vi "Keithley 2002 Multi Read.vi"(0 "GPIB address":string="16", 1 "delay (secs)":dbl min=0.0 max=999999.999 format="%.3f", 2 "source (imm:1)":u16(ring)=1 items=["hold", "immediate", "timer", "manual", "bus", "trigger link", "external"], 3 "timer value (secs)":dbl=0.001 min=0.001 max=999999.999 format="%.3f", 4 "count value":dbl=10.0 min=2.0 max=30092.0 step=1.0, 5 "error in":T2, 7 "delay between\nbus triggers (mS)":dbl=300.0 min=0.0 step=1.0) -> (6 "measurements":T1(array[cluster]) {"measurement" format="%.6e"}, 8 "error out":T2)   [LabVIEW 2020]
doc: "This VI is used to control the Measure Layer (Trigger) settings and then read back the specified number of readings.\n\nThe function of the instrument will not be changed. To take measurements for a new function, you must first configure the instrument with that function's VI.\n\nThe element of the array that stores readings is always 1 number less than the reading number. For example, the array starts at the number 0, while the readings start at 1."
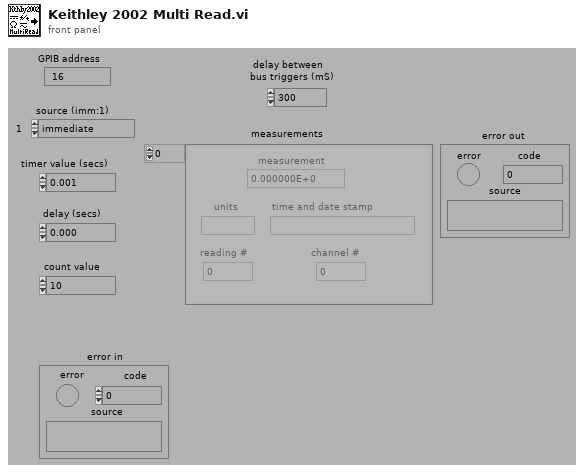
[diagram p1: front panel]
types:
  T1 = cluster{"measurement":dbl, "units":string, "time and date stamp":string, "reading #":dbl, "channel #":dbl}[]
  T2 = cluster{"error":bool, "code":i32, "source":string}
  T3 = cluster{dbl, "read buffer":string, "read buffer":string, dbl, dbl}
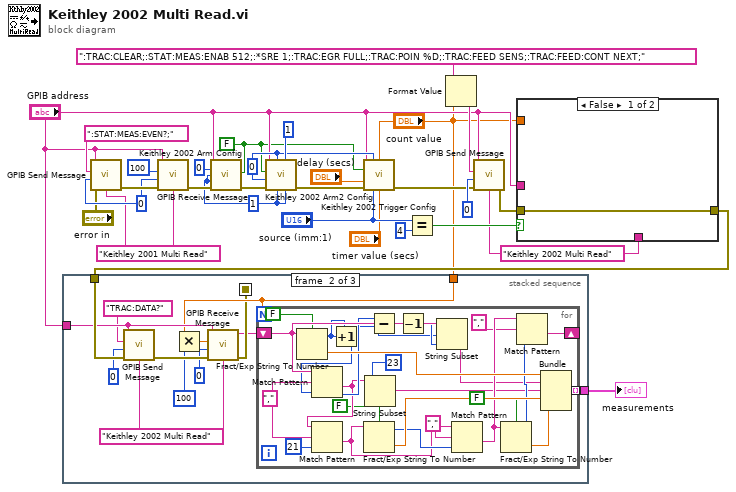
[diagram p0: block diagram]
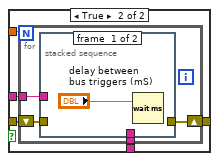
[diagram p2: hidden frame]
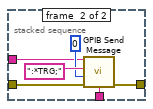
[diagram p3: hidden frame]
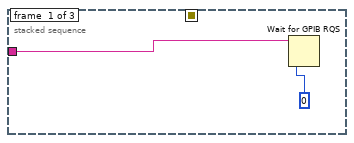
[diagram p4: hidden frame]
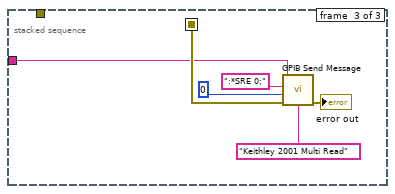
[diagram p5: hidden frame]
diagram:
  w18 = "Keithley 2001 Multi Read"
  w24 = 0
  w7 = 0
  w5 = FALSE
  w3 = 1
  w20 = "Keithley 2002 Multi Read"
  n1 = call "GPIB Send Message.vi"("address string"="GPIB address", "write buffer"=":STAT:MEAS:EVEN?;", "source"=w18, "write mode (set END:0)"=w24, "error in"="error in") -> ("error out"=w27:T2)  [unwired: 2 in, 2 out]
  n2 = call "GPIB Receive Message.vi"("address string"="GPIB address", "byte count"=100, "source"=w18, "read mode"=w24, "error in"=w27) -> ("error out"=w15:T2)  [unwired: 2 in, 2 out]
  n3 = call "Keithley 2002 Arm Config.vi"("GPIB address"="GPIB address", "count (set:0)"=0, "count value"=w3, "direction"=w5, "source (imm:1)"=w3, "error in"=w15) -> ("error out"=w14:T2)  [unwired: 9 in]
  n4 = call "Keithley 2002 Arm2 Config.vi"("timer value (secs)"=w3, "count value"=1, "source (imm:1)"=w3, "count (set:0)"=w7, "error in"=w14, "delay (secs)"=w7, "direction"=w5, "GPIB address"="GPIB address") -> ("error out"=w13:T2)  [unwired: 3 in]
  n5 = call "Keithley 2002 Trigger Config.vi"("GPIB address"="GPIB address", "count (set:0)"=w7, "count value"="count value", "direction"=w5, "delay (secs)"="delay (secs)", "error in"=w13, "source (imm:1)"="source (imm:1)", "timer value (secs)"="timer value (secs)") -> ("error out"=w12:T2)  [unwired: 7 in]
  n6 = Equal?(x="source (imm:1)", y=4) -> (x = y?=w21:bool)
  n7 = Format Value(format string=":TRAC:CLEAR;:STAT:MEAS:ENAB 512;:*SRE 1;:TRAC:EGR FULL;:TRAC:POIN %D;:TRAC:FEED SENS;:TRAC:FEED:CONT NEXT;", value (0)="count value") -> (output string=w16:string)  [unwired: 1 in]
  n8 = call "GPIB Send Message.vi"("address string"="GPIB address", "write buffer"=w16, "source"=w20, "write mode (set END:0)"=0, "error in"=w12) -> ("error out"=w22:T2)  [unwired: 2 in, 2 out]
  n9 = case shown="False" w21 {
    tunnel: [w30 w35] -> w19
    tunnel: w20 -> [_ w34]
    tunnel: "GPIB address" -> [_ w33]
    tunnel: w22 -> [w30 w32]
    tunnel: "count value" -> [_ w31]
    frame False {
    }
    frame True {
      n10 = for {
        N: w31 -> [_]
        shift-right: [w37] -> w35
        shift-left: w32 -> [w38]
        tunnel: w34 -> [w36]
        tunnel: w33 -> [w39]
        n11 = stacked-sequence {
          tunnel: w39 -> [_ w44]
          tunnel: w38 -> [_ w43]
          tunnel: [_ w42] -> w37
          tunnel: w36 -> [_ w41]
          frame #0 {
            n12 = Wait (ms)(milliseconds to wait="delay between\nbus triggers (mS)") -> ()  [unwired: 1 out]
          }
          frame #1 {
            n13 = call "GPIB Send Message.vi"("address string"=w44, "write buffer"=":*TRG;", "source"=w41, "write mode (set END:0)"=0, "error in"=w43) -> ("error out"=w42:T2)  [unwired: 2 in, 2 out]
          }
        }
      }
    }
  }
  n14 = stacked-sequence {
    seq-local: [_ w50 _] -> [_ _ w91]
    tunnel: "GPIB address" -> [w47 w59 w90]
    tunnel: w19 -> [_ w61 _]
    tunnel: [_ w52 _] -> w2
    tunnel: "count value" -> [_ w51 _]
    frame #0 {
      n15 = Wait for GPIB RQS(3:0, 4:w47) -> ()  [unwired: 1 in, 2 out]
    }
    frame #1 {
      w58 = "Keithley 2002 Multi Read"
      n16 = call "GPIB Send Message.vi"("address string"=w59, "write buffer"="TRAC:DATA?", "source"=w58, "write mode (set END:0)"=0, "error in"=w61) -> ("error out"=w60:T2)  [unwired: 2 in, 2 out]
      n17 = Multiply(x=w51, y=100) -> (x*y=w53:dbl)
      n18 = call "GPIB Receive Message.vi"("address string"=w59, "byte count"=w53, "source"=w58, "read mode"=0, "error in"=w60) -> ("read buffer"=w49:string, "error out"=w50:T2)  [unwired: 2 in, 1 out]
      n19 = for {
        N: w51 -> [_]
        shift-right: [w77] -> _
        shift-left: w49 -> [w76]
        tunnel: [w65] -> w52 mode=indexing
        w82 = ","
        n20 = Fract/Exp String To Number(use system decimal point (T)=FALSE, string=w76) -> (offset past number=w70:i32, number=w87:dbl)  [unwired: 2 in]
        n21 = Increment(x=w70) -> (x+1=w71:i32)
        n22 = Match Pattern(string=w76, regular expression=w82, offset (0)=w71) -> (after substring=w69:string, offset past match=w74:i32)  [unwired: 2 out]
        n23 = Match Pattern(string=w69, regular expression=w82, offset (0)=21) -> (after substring=w83:string)  [unwired: 3 out]
        n24 = Fract/Exp String To Number(use system decimal point (T)=FALSE, string=w83) -> (offset past number=w84:i32, number=w86:dbl)  [unwired: 2 in]
        n25 = String Subset(string=w69, length (rest)=23) -> (substring=w68:string)  [unwired: 1 in]
        n26 = Subtract(x=w74, y=w70) -> (x-y=w75:i32)
        n27 = Decrement(x=w75) -> (x-1=w72:i32)
        n28 = String Subset(string=w76, offset (0)=w70, length (rest)=w72) -> (substring=w73:string)
        n29 = Match Pattern(string=w83, regular expression=",", offset (0)=w84) -> (after substring=w80:string)  [unwired: 3 out]
        n30 = Fract/Exp String To Number(use system decimal point (T)=FALSE, string=w80) -> (offset past number=w79:i32, number=w85:dbl)  [unwired: 2 in]
        n31 = Match Pattern(string=w80, regular expression=",", offset (0)=w79) -> (after substring=w77:string)  [unwired: 3 out]
        n32 = Bundle(w87, "read buffer"=w73, "read buffer"=w68, w86, w85) -> (w65:T3)  [unwired: 1 in]
      }
    }
    frame #2 {
      n33 = call "GPIB Send Message.vi"("address string"=w90, "write buffer"=":*SRE 0;", "source"="Keithley 2001 Multi Read", "write mode (set END:0)"=0, "error in"=w91) -> ("error out"=→"error out":T2)  [unwired: 2 in, 2 out]
    }
  }
  "measurements" <- w2
